vi "DrawShots.vi"(7 "Clear":bool, 10 "IntensityArray_IN":u8[][](array[numeric]), 11 "Shot":T1) -> (2 "IntensityArray_OUT":u8[][](array[numeric]), 3 "Shot_OUT":T1)   [LabVIEW 2022 SP3]
uses:
  ShotCluster.ctl
  move_dir_ud.ctl
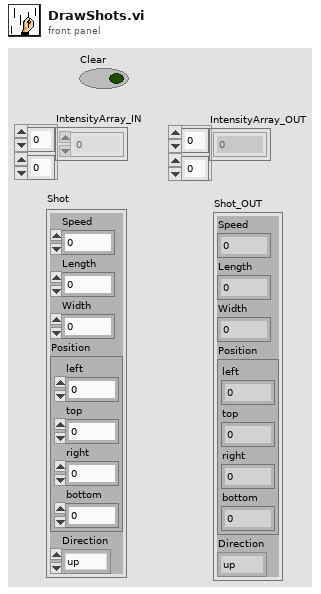
[diagram p1: front panel]
types:
  T1 = typedef "ShotCluster.ctl" = cluster{"Speed":u32, "Length":u32, "Width":u32, "Position":cluster{"left":i16, "top":i16, "right":i16, "bottom":i16}, "Direction":T2}
  T2 = typedef "move_dir_ud.ctl" = enum16{"up", "down"}
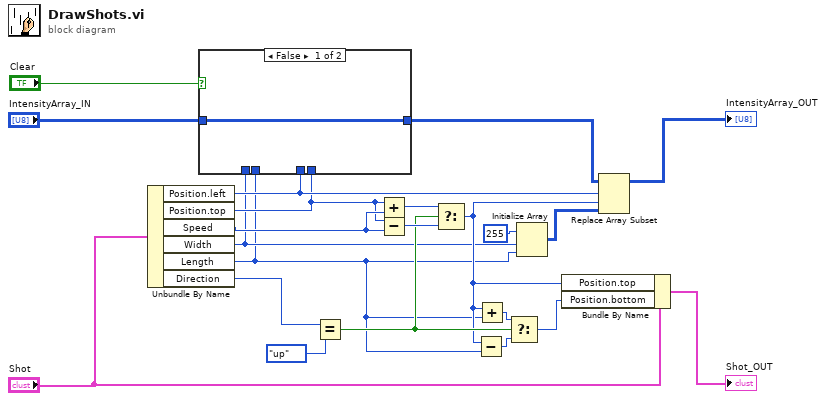
[diagram p0: block diagram]
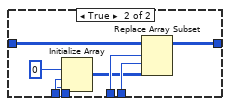
[diagram p2: hidden frame]
diagram:
  n1 = Unbundle By Name("Shot") -> ("Position.left"=w5:i16, "Position.top"=w4:i16, "Speed"=w10:u32, "Width"=w3:u32, "Length"=w1:u32, "Direction"=w22:T2)
  n2 = case shown="False" "Clear" {
    tunnel: [w23 w31] -> w7
    tunnel: "IntensityArray_IN" -> [w23 w30]
    tunnel: w5 -> [_ w29]
    tunnel: w4 -> [_ w28]
    tunnel: w3 -> [_ w25]
    tunnel: w1 -> [_ w24]
    frame False {
    }
    frame True {
      n3 = Initialize Array(u32 0 ("element"), w25, w24) -> (w27:u32[][])
      n4 = Replace Array Subset(array=w30, new element=w27, index (row)=w29, index (col)=w28) -> (w31:u8[][])
    }
  }
  n5 = Equal?(x=w22, y=move_dir_ud."up" ("Direction")) -> (x = y?=w15:bool)
  n6 = Add(x=w4, y=w10) -> (x+y=w17:u32)
  n7 = Subtract(x=w4, y=w10) -> (x-y=w16:u32)
  n8 = Select(t=w17, s=w15, f=w16) -> (s? t:f=w11:u32)
  n9 = Subtract(x=w11, y=w1) -> (x-y=w13:u32)
  n10 = Add(x=w11, y=w1) -> (x+y=w14:u32)
  n11 = Select(t=w14, s=w15, f=w13) -> (s? t:f=w12:u32)
  n12 = Initialize Array(u32 255 ("element"), w3, w1) -> (w19:u32[][])
  n13 = Bundle By Name(cluster="Shot", "Position.top"=w11, "Position.bottom"=w12) -> (→"Shot_OUT":T1)
  n14 = Replace Array Subset(array=w7, new element=w19, index (row)=w5, index (col)=w11) -> (→"IntensityArray_OUT":u8[][])
